vi "UDCUtilityGetLibraryPath.vi"() -> (3 "Library Path":path)   [LabVIEW 2020, in "niceiplib.lvlib"]
uses:
  <vilib>/UDC/niceiplib.lvlib
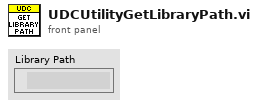
[diagram p1: front panel]
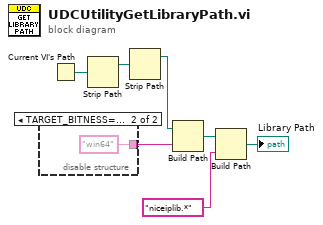
[diagram p0: block diagram]
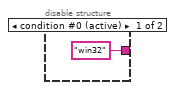
[diagram p2: hidden frame]
diagram:
  n1 = disable-structure shown="TARGET_BITNESS==64" {
    disable-tunnel: ["win32" ("name or relative path") "win64" ("name or relative path")] -> w6
    frame condition #0 (active) {
    }
    frame condition #1 {
    }
  }
  n2 = Current VI's Path() -> (path=w3:path)
  n3 = Strip Path(path=w3) -> (stripped path=w4:path)  [unwired: 1 out]
  n4 = Strip Path(path=w4) -> (stripped path=w5:path)  [unwired: 1 out]
  n5 = Build Path(base path=w5, name or relative path=w6) -> (appended path=w7:path)
  n6 = Build Path(base path=w7, name or relative path="niceiplib.*") -> (appended path=→"Library Path":path)
